vi "Parameter is settable on fly or is settable.vi"(0 "AllCameraParameters":T1[](array[typedef]), 5 "Name":string) -> (4 "SettableOnFly?":bool, 6 "Settable?":bool, 10 "SettableOnLive?":bool)   [LabVIEW 2020]
uses:
  ParameterID.ctl
  CameraParameters_Type.ctl
  CameraParameters_Authorization.ctl
  CameraParameters_OnFlyAuthorization.ctl
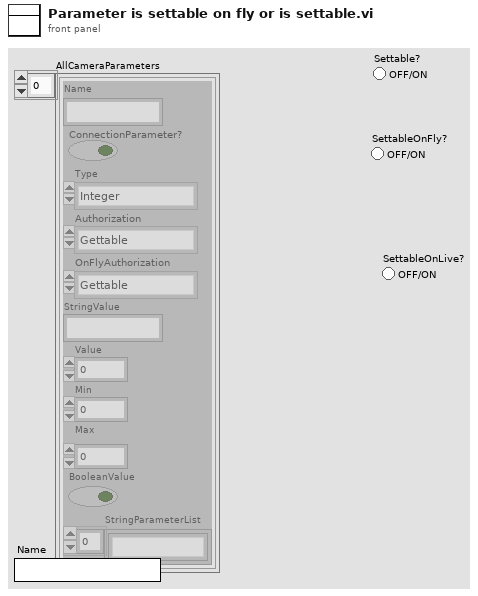
[diagram p1: front panel]
types:
  T1 = typedef "ParameterID.ctl" = cluster{"Name":string, "ConnectionParameter?":bool, "Type":T2, "Authorization":T3, "OnFlyAuthorization":T4, "StringValue":string, "Value":dbl, "Min":dbl, "Max":dbl, "BooleanValue":bool, "StringParameterList":string[]}
  T2 = typedef "CameraParameters_Type.ctl" = enum16{"Integer", "Real", "String", "Boolean"}
  T3 = typedef "CameraParameters_Authorization.ctl" = enum16{"Disable", "Gettable", "Settable - Gettable"}
  T4 = typedef "CameraParameters_OnFlyAuthorization.ctl" = enum16{"None", "Gettable", "Settable", "Settable - Gettable"}
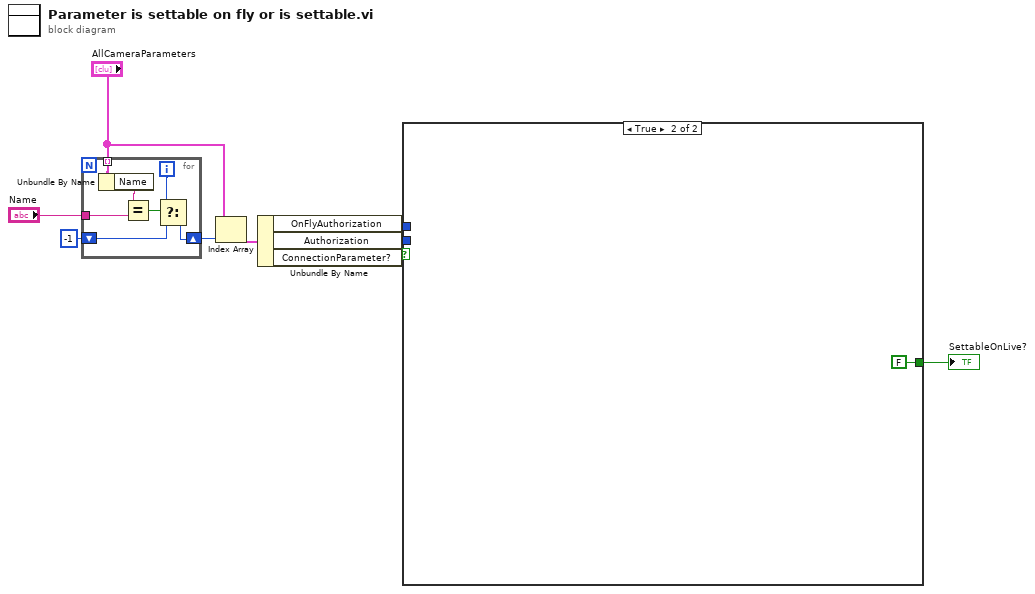
[diagram p0: block diagram]
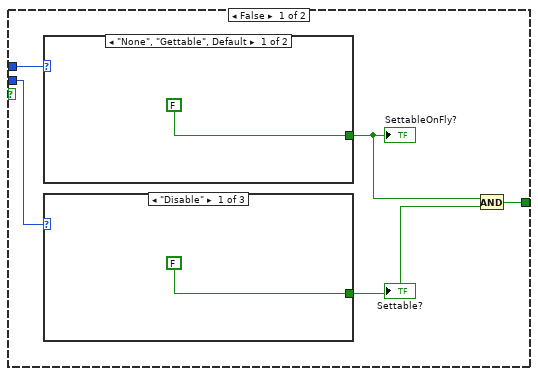
[diagram p2: hidden frame]
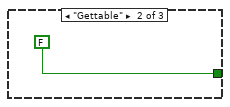
[diagram p3: hidden frame]
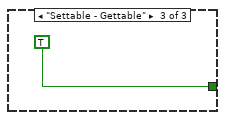
[diagram p4: hidden frame]
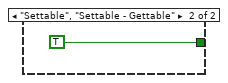
[diagram p5: hidden frame]
diagram:
  n1 = for {
    shift-right: [w14] -> w6
    shift-left: -1 -> [w13]
    tunnel: "AllCameraParameters" -> [w12] mode=indexing
    tunnel: "Name" -> [w10]
    i -> [w15]
    n2 = Unbundle By Name(w12) -> ("Name"=w11:string)
    n3 = Equal?(x=w11, y=w10) -> (x = y?=w16:bool)
    n4 = Select(t=w15, s=w16, f=w13) -> (s? t:f=w14:i32)
  }
  n5 = Index Array(array="AllCameraParameters", index=w6) -> (element=w8:T1)
  n6 = Unbundle By Name(w8) -> ("OnFlyAuthorization"=w4:T4, "Authorization"=w3:T3, "ConnectionParameter?"=w1:bool)
  n7 = case shown="True" w1 {
    tunnel: w4 -> [w21 _]
    tunnel: w3 -> [w20 _]
    tunnel: [w17 FALSE] -> w2
    frame False {
      n8 = case shown="\"None\", \"Gettable\", Default" w21 {
        tunnel: [FALSE TRUE] -> w19
        frame "None", "Gettable", Default {
        }
        frame "Settable", "Settable - Gettable" {
        }
      }
      "SettableOnFly?" <- w19
      n9 = case shown="\"Disable\"" w20 {
        tunnel: [FALSE FALSE TRUE] -> w18
        frame "Disable" {
        }
        frame "Gettable" {
        }
        frame "Settable - Gettable" {
        }
      }
      "Settable?" <- w18
      n10 = And(x=w19, y=w18) -> (x .and. y?=w17:bool)
    }
    frame True {
    }
  }
  "SettableOnLive?" <- w2
